vi "SeimensS7Net_ReadInt16[].vi"(8 "error in (no error)":errorcluster caption="错误输入（无错误）", 9 "length":u16=1000, 10 "address":string="DB600.0", 11 "Seimens 输入":refnum<class "Seimens.lvclass">) -> (0 "error out":errorcluster caption="错误输出", 2 "ReadArray":i16[](array[numeric]), 3 "Seimens 输出":refnum<class "Seimens.lvclass">)   [LabVIEW 2018, in "Seimens.lvclass"]
uses:
  Seimens.lvclass
  Seimens.lvclass/Seimens.ctl
  D:/LiMing/Labview/lib/LM_HslCommunication/DLL/HslCommunication.dll
  DLL/HslCommunication.dll
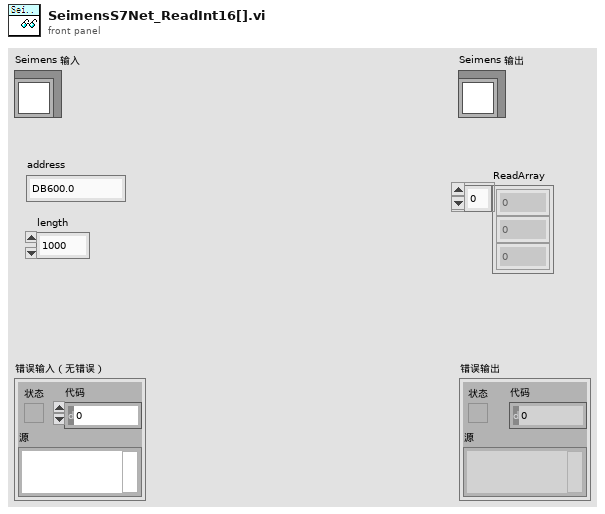
[diagram p1: front panel]
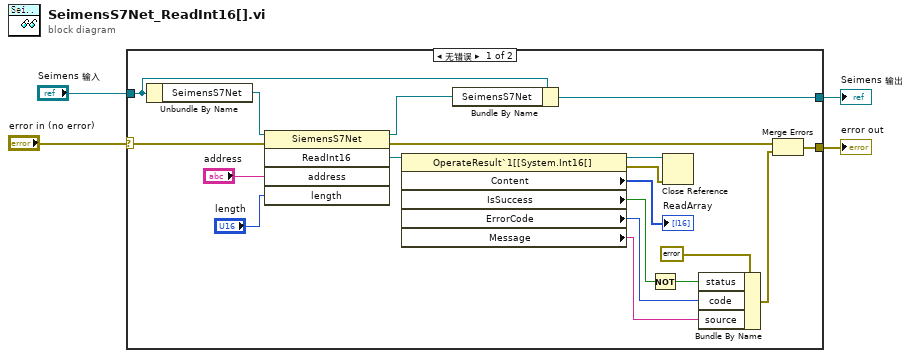
[diagram p0: block diagram]
diagram:
  n1 = case shown="无错误" "error in (no error)" {
    selector: "error in (no error)" -> [w7 w25]
    tunnel: [w6 w25] -> w3
    tunnel: [w9 w24] -> w1
    tunnel: "Seimens 输入" -> [w10 w24]
    frame No Error {
      n2 = Unbundle By Name(w10) -> ("SeimensS7Net"=w11:refnum<k24>)
      n3 = invoke class="SiemensS7Net" method="ReadInt16"(reference=w11, error in=w7, "address"="address", "length"="length") -> (reference out=w8:refnum<k24>, error out=w18:errorcluster, "ReadInt16"=w15:refnum<k24>)  [unwired: 1 in, 2 out]
      n4 = property class="OperateResult`1[[System.Int16[]"(reference=w15) -> (reference out=w17:refnum<k24>, error out=w16:errorcluster, "Content"=→"ReadArray":i16[], "IsSuccess"=w19:bool, "ErrorCode"=w20:i32, "Message"=w21:string)  [unwired: 1 in]
      n5 = Bundle By Name(cluster=w10, "SeimensS7Net"=w8) -> (w9:refnum<class "Seimens.lvclass">)
      n6 = Not(x=w19) -> (.not. x?=w5:bool)
      n7 = Close Reference(reference=w17, error in (no error)=w16) -> ()  [unwired: 1 out]
      n8 = Bundle By Name(cluster=errorcluster {"status"=FALSE, "code"=0, "source"=""} ("error in (no error)"), "status"=w5, "code"=w20, "source"=w21) -> (w22:errorcluster)
      n9 = Merge Errors(w18, w22) -> (w6:errorcluster)
    }
    frame Error {
    }
  }
  "error out" <- w3
  "Seimens 输出" <- w1
